vi "set_electrodes (SubVI).vi"(0 "Tot Electrode Arr":dbl[](array[numeric]), 5 "electrodes task 2":refnum<k21>, 9 "electrodes error":errorcluster, 11 "electrodes reference":refnum<vi>, 12 "Num samples":i32) -> (4 "electrode arr":dbl[][](array[numeric]), 6 "electrodes task":refnum<k21>, 10 "DC volts arr":dbl[](array[numeric]), 13 "Use arbitrary\nforce func?":bool, 14 "Electrode to sweep:":i32, 15 "electrodes task error":errorcluster)   [LabVIEW 2014]
uses:
  <vilib>/Utility/file.llb/Read From Spreadsheet File (DBL).vi
  <resource>/objmgr/daqmx.rc
  <vilib>/measure/NI_MABase.lvlib
panel:
  out "SampClk.Rate":dbl
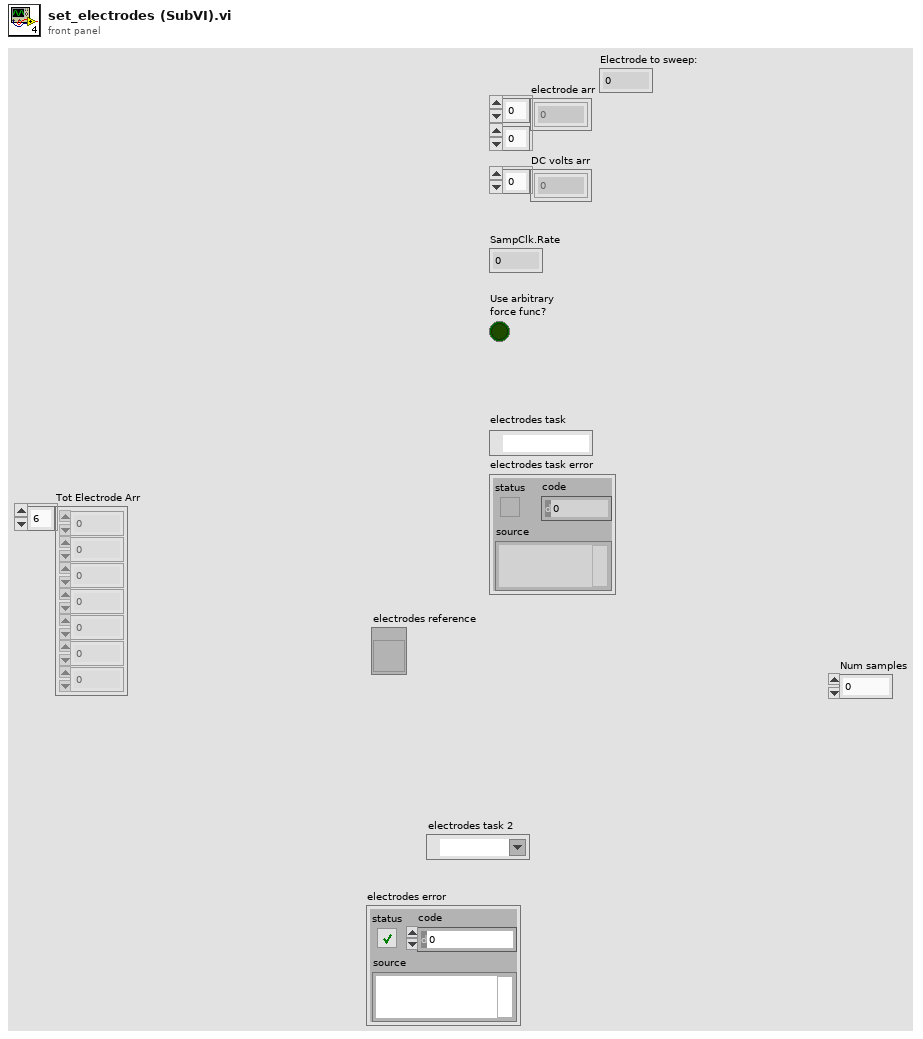
[diagram p1: front panel]
types:
  T1 = cluster{"DC volts (V):\n":dbl[], "Electrode to sweep:":i32, "start volt (V)":ext, "stop volt (V) ":ext, "# V Steps":i32, "start freq (Hz)":ext, "stop freq (Hz) ":ext, "# F steps":i32, "start DC (V)":ext, "stop DC (V)":ext, "# DC steps ":i32, "Digitize electrode\ndrives?":bool, "Sweep electrode?":bool, "Add 0.5*V DC \noffset for amp?":bool, "Use electrode \nconfig file?":bool, "Path":path, "Use arbitrary\nforce func?":bool, "Voltage vs pos file":path, "Use Arbitrary elec drive":bool, "Elec Drive File":path, "Filter Elecs?":bool, "Filter Cantilever?":bool}
  T2 = enum16{"Sine Wave", "Triangle Wave", "Square Wave", "Sawtooth Wave"}
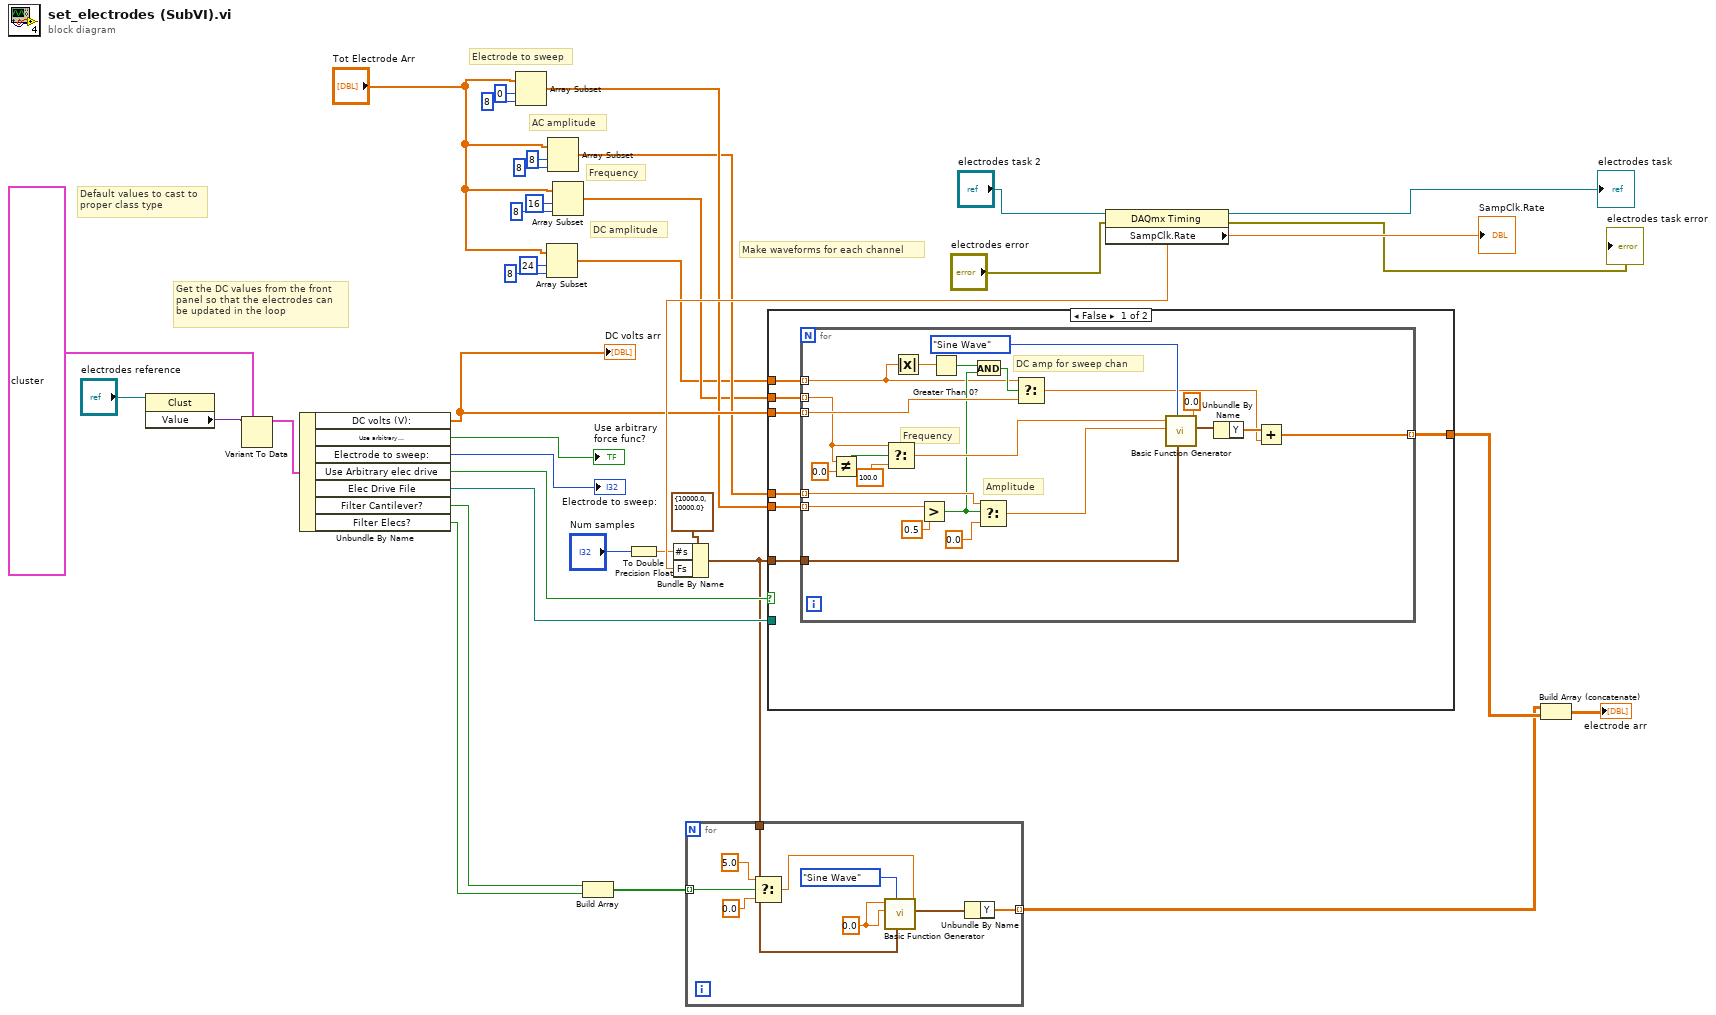
[diagram p0: block diagram]
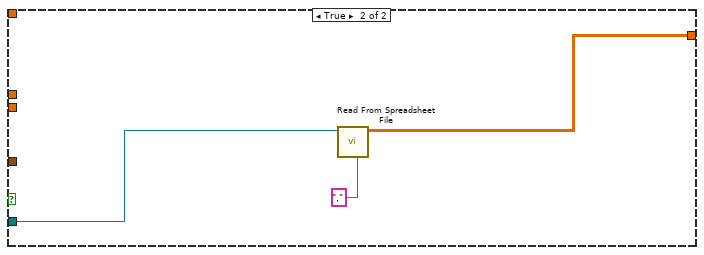
[diagram p2: hidden frame]
diagram:
  # "Default values to cast to\nproper class type"
  # "Get the DC values from the front\npanel so that the electrodes can\nbe updated in the loop"
  # "Make waveforms for each channel"
  # "DC amplitude"
  # "Frequency"
  # "AC amplitude"
  # "Electrode to sweep"
  n1 = property on="Property Node" class="Clust"(reference="electrodes reference") -> ("Value"=w30:variant)  [unwired: 1 in, 2 out]
  n2 = Variant To Data(type=T1 {"DC volts (V):\n"=[0.0, 0.0, 0.0, 0.0, 0.0, 0.0, 0.0, 0.0], "Electrode to sweep:"=3, "start volt (V)"=0.0, "stop volt (V) "=0.0, "# V Steps"=1, "start freq (Hz)"=41.0, "stop freq (Hz) "=41.0, "# F steps"=1, "start DC (V)"=0.0, "stop DC (V)"=0.0, "# DC steps "=1, "Digitize electrode\ndrives?"=TRUE, "Sweep electrode?"=FALSE, "Add 0.5*V DC \noffset for amp?"=FALSE, "Use electrode \nconfig file?"=FALSE, "Path"=path "", "Use arbitrary\nforce func?"=FALSE, "Voltage vs pos file"=path "", "Use Arbitrary elec drive"=FALSE, "Elec Drive File"=path "", "Filter Elecs?"=FALSE, "Filter Cantilever?"=FALSE} ("Electrode settings:"), Variant=w30) -> (data=w29:T1)  [unwired: 1 in, 1 out]
  n3 = Unbundle By Name(w29) -> ("DC volts (V):"=w28:dbl[], "Use arbitrary\nforce func?"=→"Use arbitrary\nforce func?":bool, "Electrode to sweep:"=→"Electrode to sweep:":i32, "Use Arbitrary elec drive"=w9:bool, "Elec Drive File"=w8:path, "Filter Cantilever?"=w6:bool, "Filter Elecs?"=w5:bool)
  "DC volts arr" <- w28
  n4 = Array Subset(array="Tot Electrode Arr", index=0, length=8) -> (w25:dbl[])
  n5 = Array Subset(array="Tot Electrode Arr", index=24, length=8) -> (w17:dbl[])
  n6 = Array Subset(array="Tot Electrode Arr", index=8, length=8) -> (w24:dbl[])
  n7 = Array Subset(array="Tot Electrode Arr", index=16, length=8) -> (w19:dbl[])
  n8 = Build Array(w6, w5) -> (w4:bool[])
  n9 = To Double Precision Float(number="Num samples") -> (double precision float=w13:dbl)
  n10 = property class="DAQmx Timing"(reference="electrodes task 2", error in="electrodes error") -> (reference out=→"electrodes task":refnum<k21>, error out=→"electrodes task error":errorcluster, "SampClk.Rate"=w34:dbl)
  "SampClk.Rate" <- w34
  n11 = Bundle By Name(cluster=cluster{"Fs":dbl, "#s":dbl} {"Fs"=10000.0, "#s"=10000.0} ("sampling info"), "#s"=w13, "Fs"=w34) -> (w7:cluster{"Fs":dbl, "#s":dbl})
  n12 = for {
    tunnel: w7 -> [w46]
    tunnel: w4 -> [w39] mode=indexing
    tunnel: [w38] -> w1 mode=indexing
    w43 = 0.0 ("f")
    n13 = Select(t=5.0 ("f"), s=w39, f=0.0) -> (s? t:f=w41:dbl)
    n14 = call <vilib>:"Basic Function Generator.vi"("offset"=w41, "sampling info"=w46, "signal type"=T2."Sine Wave", "amplitude"=w43, "frequency"=w43) -> ("signal out"=w40:waveform(dbl))  [unwired: 4 in, 2 out]
    n15 = Unbundle By Name(w40) -> ("Y"=w38:dbl[])
  }
  n16 = case shown="False" w9 {
    tunnel: w7 -> [w47 _]
    tunnel: [w53 w78] -> w2
    tunnel: w28 -> [w52 _]
    tunnel: w25 -> [w51 _]
    tunnel: w24 -> [w50 _]
    tunnel: w19 -> [w49 _]
    tunnel: w17 -> [w48 _]
    tunnel: w8 -> [_ w77]
    frame False {
      n17 = for {
        tunnel: w52 -> [w70] mode=indexing
        tunnel: w49 -> [w65] mode=indexing
        tunnel: w50 -> [w73] mode=indexing
        tunnel: w47 -> [w72]
        tunnel: [w57] -> w53 mode=indexing
        tunnel: w48 -> [w54] mode=indexing
        tunnel: w51 -> [w69] mode=indexing
        # "DC amp for sweep chan"
        # "Frequency"
        # "Amplitude"
        n18 = Not Equal?(x=w65, y=0.0) -> (x != y?=w66:bool)
        n19 = Select(t=w65, s=w66, f=100.0) -> (s? t:f=w64:dbl)
        n20 = Absolute Value(x=w54) -> (abs(x)=w55:dbl)
        n21 = Greater?(x=w69, y=0.5) -> (0:w61:bool)
        n22 = Greater Than 0?(x=w55) -> (x > 0?=w56:bool)
        n23 = And(x=w56, y=w61) -> (x .and. y?=w62:bool)
        n24 = Select(t=w73, s=w61, f=0.0) -> (s? t:f=w75:dbl)
        n25 = Select(t=w54, s=w62, f=w70) -> (s? t:f=w58:dbl)
        n26 = call <vilib>:"Basic Function Generator.vi"("offset"=0.0, "sampling info"=w72, "signal type"=T2."Sine Wave", "amplitude"=w75, "frequency"=w64) -> ("signal out"=w71:waveform(dbl))  [unwired: 4 in, 2 out]
        n27 = Unbundle By Name(w71) -> ("Y"=w59:dbl[])
        n28 = Add(x=w59, y=w58) -> (x+y=w57:dbl[])
      }
    }
    frame True {
      n29 = call-poly <vilib>:"Read From Spreadsheet File.vi"("delimiter (\\t)"=",", "file path (dialog if empty)"=w77) -> ("all rows"=w78:dbl[][])  [unwired: 5 in, 4 out]
    }
  }
  n30 = Build Array (concatenate)(w1, w2) -> (→"electrode arr":dbl[][])
